vi "Is Grave.vi"(8 "Error In":errorcluster, 11 "GObject In":refnum<vi>) -> (0 "Error Out":errorcluster, 2 "Grave?":bool, 3 "GObject Out":refnum<vi>)   [LabVIEW 2017, in "Toolkit.lvlib"]
doc: "Checks if a GObject is a grave. A grave is Diagram Disable Structure with a RIP bookmark tag for its label, a.k.a. tombstone."
uses:
  Toolkit.lvlib
  Typedefs/Bookmark Tags.ctl
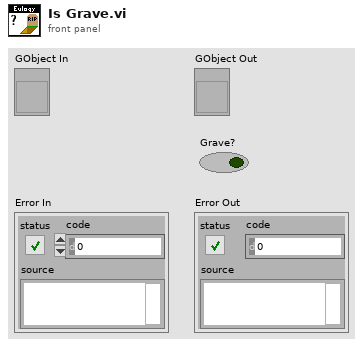
[diagram p1: front panel]
types:
  T1 = typedef "Toolkit.lvlib/Bookmark Tags.ctl" = enum16{"RIP", "Zombie"}
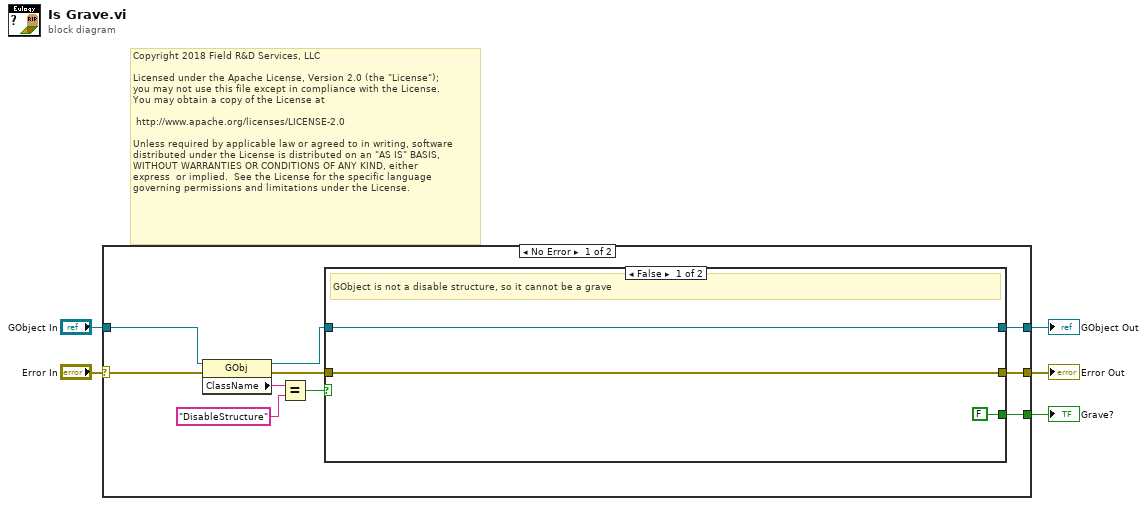
[diagram p0: block diagram]
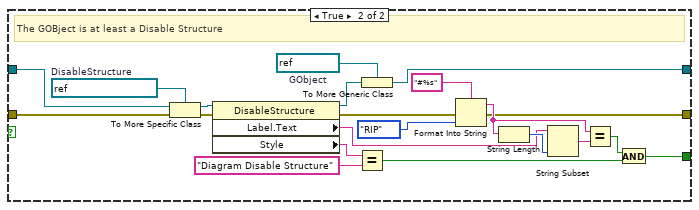
[diagram p2: hidden frame]
diagram:
  # "Copyright 2018 Field R&D Services, LLC\n\nLicensed under the Apache License, Version 2.0 (the \"License\");\nyou may not use this file except in compliance with the License.\nYou may obtain a copy of the License at\n\n\thttp://www.apache.org/licenses/LICENSE-2.0\n\nUnless required by applicable law or agreed to in writing, software\ndistributed under the License is distributed on an \"AS IS\" BASIS,\nWITHOUT WARRANTIES OR CONDITIONS OF ANY KIND, either \nexpress  or implied.  See the License for the specific language \ngoverning permissions and limitations under the License."
  n1 = case shown="No Error" "Error In" {
    selector: "Error In" -> [w6 w40]
    tunnel: "GObject In" -> [w15 w41]
    tunnel: [w14 _] -> w4
    tunnel: [w8 w40] -> w3
    tunnel: [w7 w41] -> w2
    frame No Error {
      n2 = property class="GObj"(reference=w15, error in=w6) -> (reference out=w13:refnum<vi>, error out=w12:errorcluster, "ClassName"=w11:string)
      n3 = Equal?(x=w11, y="DisableStructure") -> (x = y?=w9:bool)
      n4 = case shown="False" w9 {
        tunnel: [FALSE w28] -> w14
        tunnel: w13 -> [w16 w25]
        tunnel: w12 -> [w18 w27]
        tunnel: [w18 w22] -> w8
        tunnel: [w16 w20] -> w7
        frame False {
          # "GObject is not a disable structure, so it cannot be a grave"
        }
        frame True {
          w19 = refnum<vi> refnum  # GObject
          w23 = refnum<vi> refnum  # DisableStructure
          # "The GOBject is at least a Disable Structure"
          n5 = To More Specific Class(target class=w23, reference=w25, error in=w27) -> (specific class reference=w24:refnum<vi>, error out=w26:errorcluster)
          n6 = property class="DisableStructure"(reference=w24, error in=w26) -> (reference out=w21:refnum<vi>, error out=w33:errorcluster, "Label.Text"=w37:string, "Style"=w32:string)
          n7 = Equal?(x=w32, y="Diagram Disable Structure") -> (x = y?=w29:bool)
          n8 = To More Generic Class(target class=w19, reference=w21) -> (generic class reference=w20:refnum<vi>)
          n9 = Format Into String(format string="#%s", error in=w33, Bookmark_Tags."RIP" ("Bookmark")) -> (resulting string=w36:string, error out=w22:errorcluster)  [unwired: 1 in]
          n10 = String Length(string=w36) -> (length=w38:i32)
          n11 = String Subset(string=w37, length (rest)=w38) -> (substring=w39:string)  [unwired: 1 in]
          n12 = Equal?(x=w36, y=w39) -> (x = y?=w30:bool)
          n13 = And(x=w30, y=w29) -> (x .and. y?=w28:bool)
        }
      }
    }
    frame Error {
    }
  }
  "Grave?" <- w4
  "GObject Out" <- w2
  "Error Out" <- w3
